vi "Get Next.vi"(0 "Parallel":refnum<class "Parallel.lvclass">, 1 "Linked List Ref":refnum<data-value>, 5 "Active Unique ID":string, 9 "Active Element Index":i32, 11 "error in (no error)":errorcluster) -> (3 "Linked List Ref out":refnum<data-value>, 4 "Executioner out":refnum<class "Executioner.lvclass">, 6 "Active Unique ID out":string, 8 "Test Executive Ref out":refnum<data-value>, 10 "Active Element Index out":i32, 12 "Found":bool, 13 "Complete":bool, 14 "Stop":bool, 15 "error out":errorcluster)   [LabVIEW 2020, in "Test Executive.lvlib" / "Parallel.lvclass"]
uses:
  <vilib>/gpm_packages/@cs/test-executive/Source/Test Executive/Parallel/Parallel.lvclass
  C:/Program Files/National Instruments/LabVIEW 2020/vi.lib/gpm_packages/@cs/test-executive/Source/Test Executive/Executioner/Executioner.lvclass
  <vilib>/gpm_packages/@cs/test-executive/Source/Test Executive/Executioner/Executioner.lvclass
  <vilib>/gpm_packages/@cs/linked-list/Source/Linked List/ILinkedList/ILinked List.lvclass
  <vilib>/gpm_packages/@cs/test-executive/Source/Test Executive/ITestExecutive/ITest Executive.lvclass
  <vilib>/gpm_packages/@cs/test-executive/Source/Test Executive/Subroutine/Subroutine.lvclass
  <vilib>/gpm_packages/@cs/test-executive/Source/Test Executive/Parallel/Parallel.lvclass/Parallel.ctl
  a5be4b95-0d9b-41e3-bfec-5a8036420d1b.vi
  8b18314e-e67c-432c-86ad-0024e5e2993c.vi
  268824d3-31ba-4a5f-b617-ee820ad7408f.vi
  <vilib>/Utility/error.llb/Error Cluster From Error Code.vi
  <vilib>/gpm_packages/@cs/linked-list/Source/Linked List/Linked List Ref/Linked List Ref.lvclass
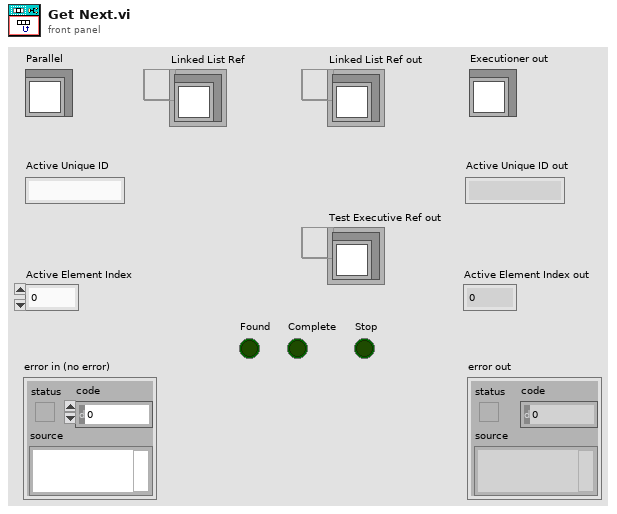
[diagram p1: front panel]
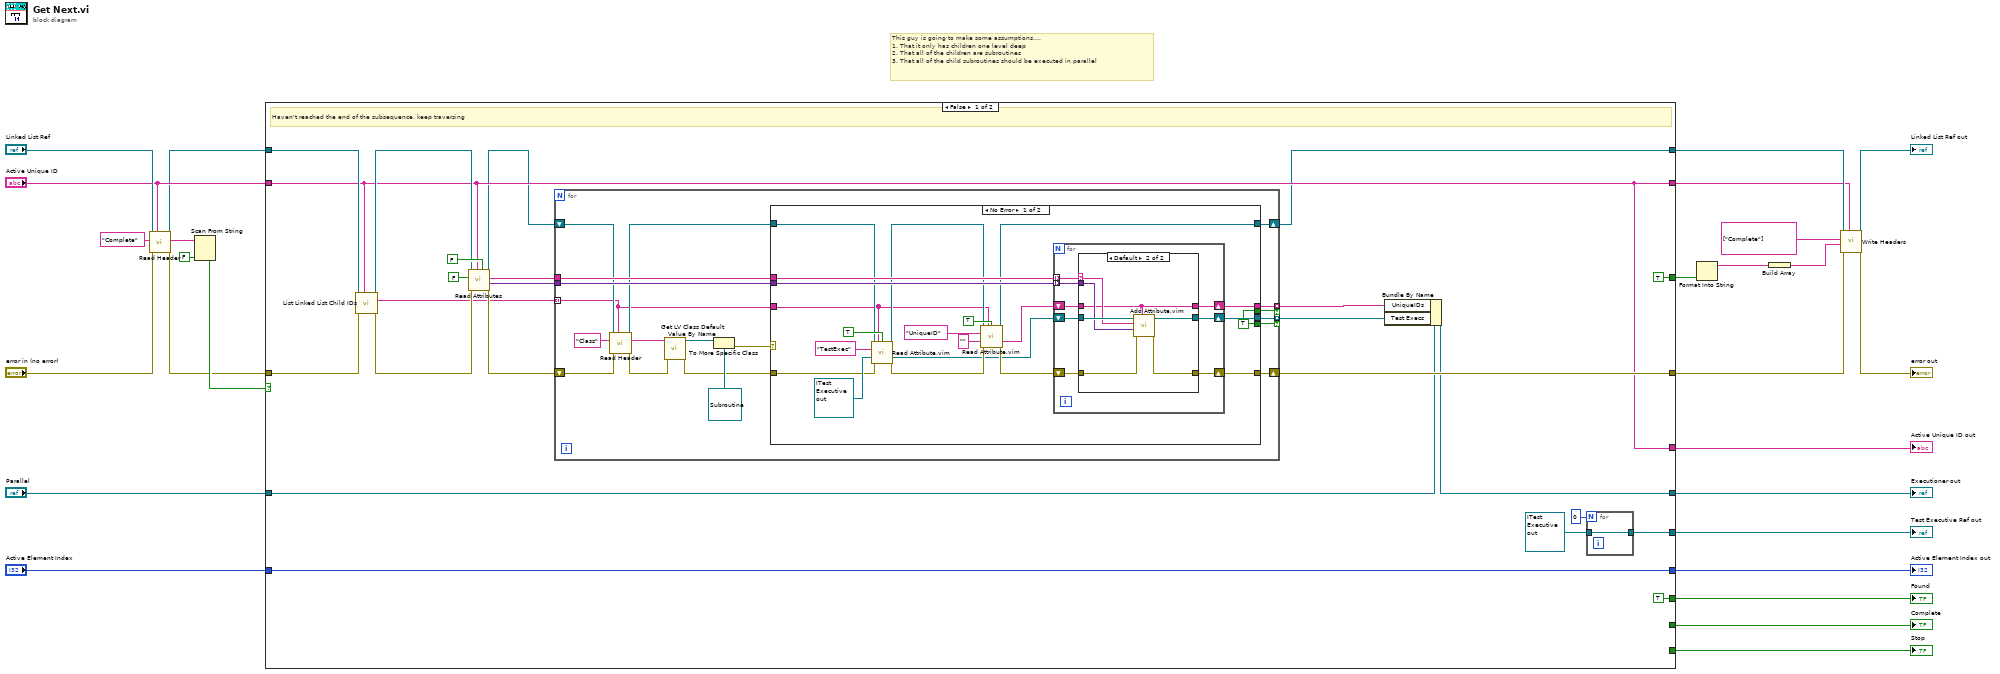
[diagram p0: block diagram]
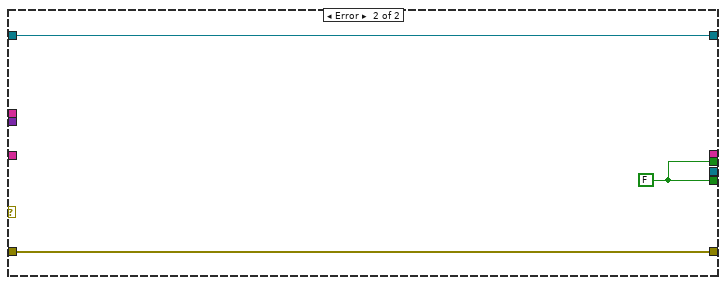
[diagram p3: hidden frame]
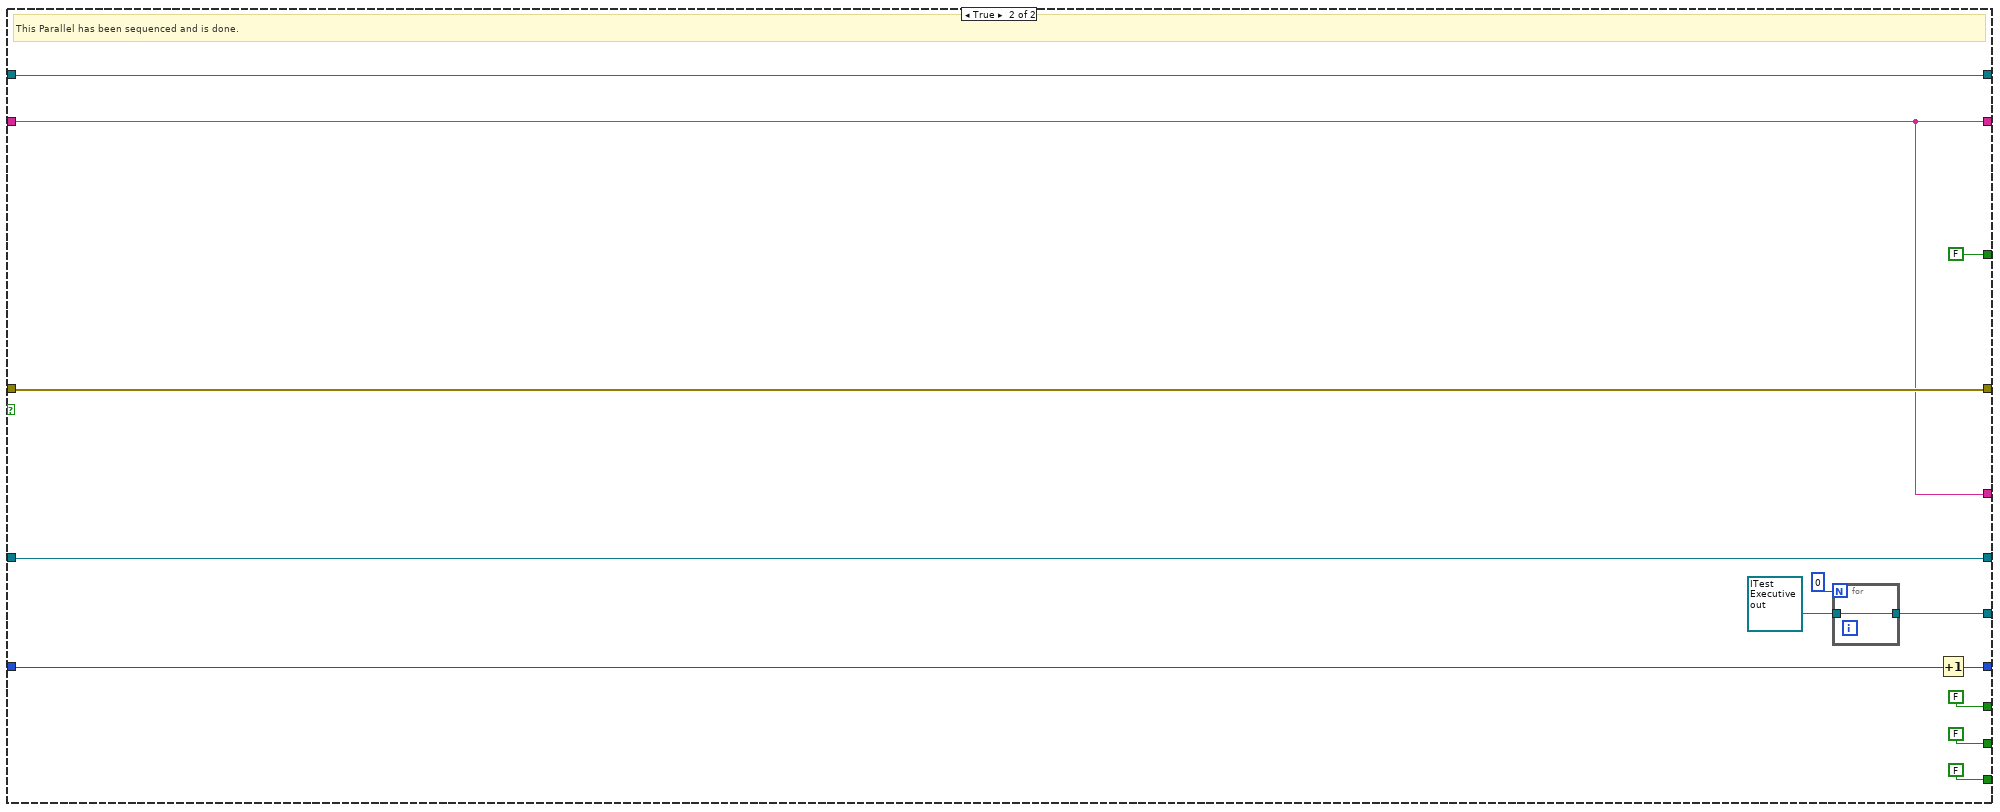
[diagram p4: hidden frame]
diagram:
  # "This guy is going to make some assumptions....\n1. That it only has children one level deep\n2. That all of the children are subroutines\n3. That all of the child subroutines should be executed in parallel"
  n1 = call <vilib>:"Read Header.vi"("Linked List ID"="Active Unique ID", "error in (no error)"="error in (no error)", "Header Name"="Complete" ("Attribute Name"), "Linked List Ref"="Linked List Ref") -> ("error out"=w1:errorcluster, "Header Value"=w5:string, "Linked List Ref out"=w2:refnum<data-value>)  [unwired: 4 in, 1 out]
  n2 = Scan From String(input string=w5, default 1=FALSE) -> (output 1=w3:bool)  [unwired: 3 in, 3 out]
  n3 = case shown="False" w3 {
    tunnel: [w28 w126] -> w13
    tunnel: w2 -> [w35 w126]
    tunnel: [w40 w125] -> w12
    tunnel: w1 -> [w33 w125]
    tunnel: "Active Element Index" -> [w51 w123]
    tunnel: [w31 w118] -> w11
    tunnel: "Active Unique ID" -> [w31 w118]
    tunnel: [w36 w124] -> w23
    tunnel: "Parallel" -> [w39 w124]
    tunnel: [w51 w122] -> w20
    tunnel: [TRUE FALSE] -> w17
    tunnel: [_ FALSE] -> w18
    tunnel: [_ FALSE] -> w19
    tunnel: [w31 w118] -> w22
    tunnel: [TRUE FALSE] -> w10
    tunnel: [w46 w114] -> w21
    frame False {
      # "Haven't reached the end of the subsequence, keep traversing"
      n4 = call <vilib>:"List Linked List Child IDs.vi"("Linked List ID"=w31, "error in (no error)"=w33, "Linked List Ref"=w35) -> ("error out"=w32:errorcluster, "Child IDs"=w30:string[], "Linked List Ref out"=w34:refnum<data-value>)  [unwired: 6 in]
      n5 = call <vilib>:"Read Attributes.vi"("Flatten Pointer?"=FALSE, "Linked List ID"=w31, "error in (no error)"=w32, "Include Private?"=FALSE, "Linked List Ref"=w34) -> ("error out"=w44:errorcluster, "Attributes"=w41:variant[], "Attribute Names out"=w43:string[], "Linked List Ref out"=w29:refnum<data-value>)  [unwired: 1 in, 2 out]
      n6 = for {
        tunnel: w43 -> [w70]
        tunnel: w41 -> [w69]
        shift-right: [w68] -> w40
        shift-left: w44 -> [w63]
        tunnel: [w67] -> w38 mode=indexing if=w53
        tunnel: [w66] -> w37 mode=indexing if=w52
        tunnel: w30 -> [w56] mode=indexing
        shift-right: [w57] -> w28
        shift-left: w29 -> [w64]
        n7 = call <vilib>:"Read Header.vi"("Linked List ID"=w56, "error in (no error)"=w63, "Header Name"="Class", "Linked List Ref"=w64) -> ("error out"=w61:errorcluster, "Header Value"=w62:string, "Linked List Ref out"=w58:refnum<data-value>)  [unwired: 4 in, 1 out]
        n8 = call <vilib>:"Get LV Class Default Value By Name.vi"("error in (no error)"=w61, "class name"=w62) -> ("error out"=w55:errorcluster, "object"=w60:refnum<class>)  [unwired: 8 in]
        n9 = To More Specific Class(target class=refnum<class "Subroutine.lvclass"> refnum ("Test Executive.lvlib:Subroutine.lvclass"), reference=w60) -> (error out=w54:errorcluster)  [unwired: 1 in, 1 out]
        n10 = case shown="No Error" w54 {
          tunnel: w70 -> [w91 _]
          tunnel: w69 -> [w90 _]
          tunnel: [w89 w111] -> w68
          tunnel: [w88 _] -> w67
          tunnel: [w87 _] -> w66
          tunnel: w58 -> [w79 w112]
          tunnel: [w77 w112] -> w57
          tunnel: w56 -> [w76 _]
          tunnel: w55 -> [w75 w111]
          tunnel: [w71 w110] -> w53
          tunnel: [w71 w110] -> w52
          frame No Error {
            w71 = TRUE
            n11 = call "Read Attribute.vim"("Linked List Ref"=w79, "Linked List ID"=w76, "Include Private?"=TRUE, "Attribute Name"="TestExec", "Type"=refnum<data-value> refnum ("Test Executive Ref out"), "error in (no error)"=w75) -> ("Linked List Ref out"=w78:refnum<data-value>, "Attribute"=w72:refnum<data-value>, "error out"=w82:errorcluster)  [unwired: 4 in, 3 out]
            n12 = call "Read Attribute.vim"("Linked List Ref"=w78, "Linked List ID"=w76, "Include Private?"=TRUE, "Attribute Name"="UniqueID", "Type"="", "error in (no error)"=w82) -> ("Linked List Ref out"=w77:refnum<data-value>, "Attribute"=w73:string, "error out"=w74:errorcluster)  [unwired: 4 in, 3 out]
            n13 = for {
              shift-right: [w96] -> w89
              shift-left: w74 -> [w97]
              tunnel: w91 -> [w95] mode=indexing
              tunnel: w90 -> [w94] mode=indexing
              shift-right: [w93] -> w88
              shift-left: w73 -> [w98]
              shift-right: [w92] -> w87
              shift-left: w72 -> [w99]
              n14 = case shown="Default" w95 {
                selector: w95 -> [_ w106]
                tunnel: w99 -> [w100 w109]
                tunnel: w98 -> [w101 w104]
                tunnel: w97 -> [w102 w108]
                tunnel: [w102 w107] -> w96
                tunnel: w94 -> [_ w105]
                tunnel: [w101 w104] -> w93
                tunnel: [w100 w103] -> w92
                frame "Restore Point" {
                }
                frame Default {
                  n15 = call "Add Attribute.vim"("ID"=w104, "error in (no error)"=w108, "Attribute"=w105, "Attribute Name"=w106, "Test Executive Ref"=w109) -> ("error out"=w107:errorcluster, "Test Executive Ref out"=w103:refnum<data-value>)  [unwired: 3 in, 2 out]
                }
              }
            }
          }
          frame Error {
            w110 = FALSE
          }
        }
      }
      n16 = Bundle By Name(cluster=w39, "UniqueIDs"=w38, "Test Execs"=w37) -> (w36:refnum<class "Parallel.lvclass">)
      n17 = for {
        N: 0 -> [_]
        tunnel: refnum<data-value> refnum ("Test Executive Ref out") -> [w113]
        tunnel: [w113] -> w46
      }
    }
    frame True {
      # "This Parallel has been sequenced and is done."
      n18 = for {
        N: 0 -> [_]
        tunnel: refnum<data-value> refnum ("Test Executive Ref out") -> [w127]
        tunnel: [w127] -> w114
      }
      n19 = Increment(x=w123) -> (x+1=w122:i32)
    }
  }
  "Executioner out" <- w23
  "Active Unique ID out" <- w22
  "Active Element Index out" <- w20
  "Found" <- w17
  "Complete" <- w18
  "Stop" <- w19
  "Test Executive Ref out" <- w21
  n20 = Format Into String(w10) -> (resulting string=w8:string)  [unwired: 3 in, 1 out]
  n21 = Build Array(w8) -> (w7:string[])
  n22 = call <vilib>:"Write Headers.vi"("Linked List ID"=w11, "error in (no error)"=w12, "Header Values"=w7, "Header Names"=string[] ["Complete"], "Linked List Ref"=w13) -> ("error out"=→"error out":errorcluster, "Linked List Ref out"=→"Linked List Ref out":refnum<data-value>)  [unwired: 5 in]
